vi "SutterController.vi"() -> ()   [LabVIEW 2012]
uses:
  <vilib>/Math Plots/3D Math Plots/3D Scatter/3D Scatter XCtrl/3D Scatter.xctl
  SerialController/Serial Controller.lvclass
  SerialController/Joystick.lvclass
  <vilib>/Utility/file.llb/Read From Spreadsheet File (DBL).vi
  <vilib>/Utility/file.llb/Write To Spreadsheet File (DBL).vi
panel:
  out "error out":errorcluster
  in  "Z limit":bool
  in  "TopLens":bool
  in  "overide":bool
  out "OutOfRange":bool
  in  "Set Maximum":bool
  in  "Set Minimum":bool
  out "positionLimits":dbl[][](array[numeric])
  out "Coarse":bool
  out "Locked":bool
  out "AxisStep":dbl[](array[numeric])
  out "ExternalInput":bool
  out "3D Scatter":refnum<class "3D Plot Datatype.lvclass">[](xcontrol)
  out "Moving":bool
  in  "stop":bool
  in  "Current Position":dbl[](array[numeric])
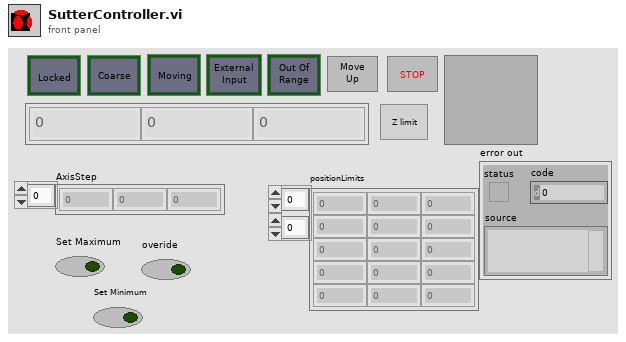
[diagram p1: front panel]
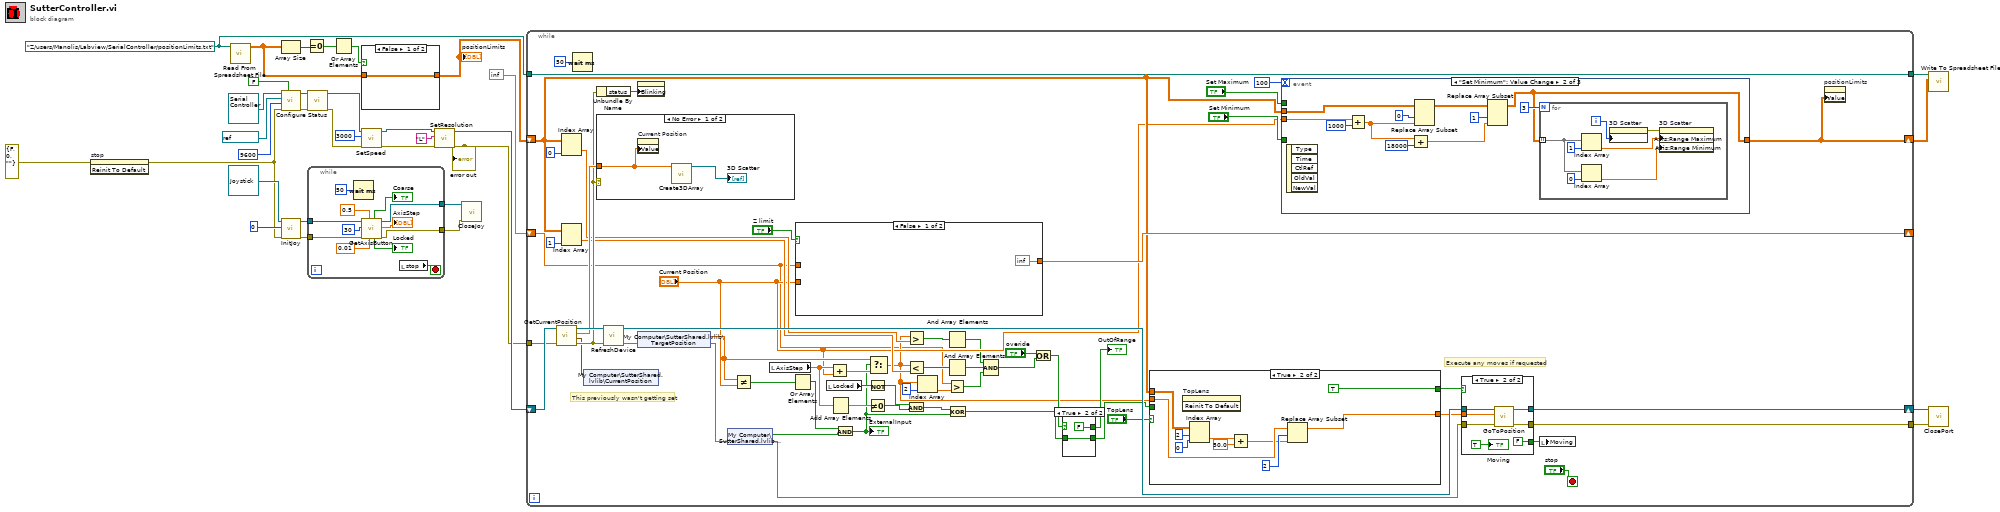
[diagram p0: block diagram]
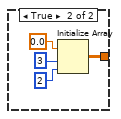
[diagram p2: hidden frame]
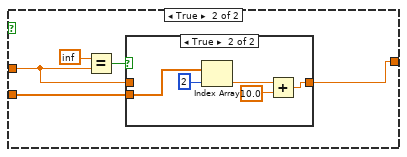
[diagram p3: hidden frame]
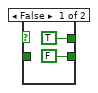
[diagram p6: hidden frame]
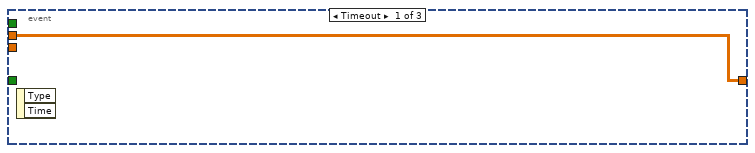
[diagram p7: hidden frame]
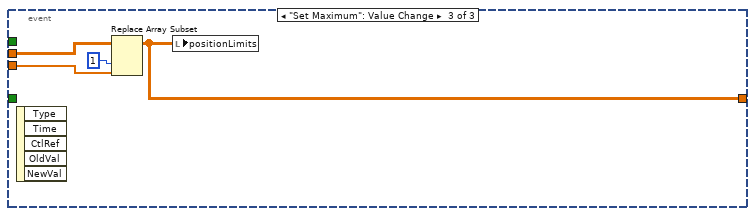
[diagram p8: hidden frame]
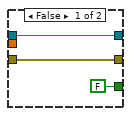
[diagram p9: hidden frame]
diagram:
  w10 = path "Z:/users/Manolis/Labview/SerialController/positionLimits.txt" ("Path")
  n1 = invoke on="stop" class="Bool (strict)" method="Reinit To Default"(error in=errorcluster {"status"=FALSE, "code"=0, "source"=""} ("error in (no error)")) -> (error out=w11:errorcluster)  [unwired: 2 in, 2 out]
  n2 = call-poly <vilib>:"Read From Spreadsheet File.vi"("file path (dialog if empty)"=w10) -> ("all rows"=w5:dbl[][])  [unwired: 6 in, 4 out]
  n3 = Array Size(array=w5) -> (size(s)=w7:i32[])
  n4 = call-dynamic "Configure.vi"("Reset"=FALSE, "error in (no error)"=w11, "baud rate (9600)"=u32 9600, "VISA resource name"=refnum<visa-resource-name> "COM6", "Serial Controller in"=refnum<class "Serial Controller.lvclass"> refnum) -> ("error out"=w32:errorcluster, "Serial Controller out"=w33:refnum<class "Serial Controller.lvclass">)  [unwired: 5 in]
  n5 = call-dynamic "InitJoy.vi"("error in (no error)"=w11, "device index"=0, "Joystick in"=refnum<class "Joystick.lvclass"> refnum) -> ("error out"=w15:errorcluster, "Joystick out"=w16:refnum<class "Joystick.lvclass">)  [unwired: 7 in]
  n6 = Equal To 0?(x=w7) -> (x = 0?=w6:bool[])
  n7 = call-dynamic "Status.vi"("error in (no error)"=w32, "Serial Controller in"=w33) -> ("error out"=w19:errorcluster, "Serial Controller out"=w21:refnum<class "Serial Controller.lvclass">)  [unwired: 7 in, 1 out]
  n8 = while {
    tunnel: w16 -> [w43]
    tunnel: w15 -> [w42]
    tunnel: [w40] -> w14
    tunnel: [w39] -> w13
    stop <- w45 stop-if-true
    n9 = Wait (ms)(milliseconds to wait=u32 50) -> ()  [unwired: 1 out]
    n10 = call-dynamic "GetAxisButton"("coarseFactor"=0.01, "fastFactor"=0.5, "error in (no error)"=w42, "timeout(s)"=u32 30, "Joystick in"=w43) -> ("error out"=w39:errorcluster, "AxisStep"=→"AxisStep":dbl[], "Joystick out"=w40:refnum<class "Joystick.lvclass">, "lock"=→"Locked":bool, "Coarse"=→"Coarse":bool)  [unwired: 2 in]
    n11 = local read "stop"() -> (w45:bool)
  }
  n12 = Or Array Elements(Boolean array=w6) -> (logical OR=w3:bool)
  n13 = case shown="False" w3 {
    tunnel: w5 -> [w46 _]
    tunnel: [w46 w47] -> w4
    frame False {
    }
    frame True {
      n14 = Initialize Array(0.0 ("element"), 3 ("dimension size"), 2 ("dimension size")) -> (w47:dbl[][])
    }
  }
  "positionLimits" <- w4
  n15 = call-dynamic "SetSpeed.vi"("error in (no error)"=w19, "Input: Speed in microns/sec"=3000, "Serial Controller in"=w21) -> ("error out"=w24:errorcluster, "Serial Controller out"=w23:refnum<class "Serial Controller.lvclass">)  [unwired: 5 in, 2 out]
  n16 = call-dynamic "SetResolution.vi"("error in (no error)"=w24, "Input: Resolution - H/L"="L", "Serial Controller in"=w23) -> ("error out"=w1:errorcluster, "Serial Controller out"=w20:refnum<class "Serial Controller.lvclass">)  [unwired: 7 in]
  "error out" <- w1
  n17 = call-dynamic "CloseJoy.vi"("error in (no error)"=w13, "Joystick in"=w14) -> ()  [unwired: 9 in, 1 out]
  n18 = while {
    shift-right: [w100] -> w27
    shift-left: w20 -> [w109]
    tunnel: [w89] -> w26
    tunnel: w1 -> [w95]
    tunnel: w10 -> [w80]
    tunnel: [w80] -> w9
    shift-right: [w65] -> w8
    shift-left: w4 -> [w62]
    shift-right: [w63] -> _
    shift-left: inf -> [w58]
    stop <- "stop" stop-if-true
    # "Execute any moves if requested"
    # "This previously wasn't getting set"
    n19 = call-dynamic "GetCurrentPosition.vi"("error in (no error)"=w95, "Serial Controller in"=w109) -> ("error out"=w105:errorcluster, "PositionBundle"=w52:cluster{"X":dbl, "Y":dbl, "Z":dbl, "Depth":dbl}, "Position"=w106:dbl[], "Serial Controller out"=w107:refnum<class "Serial Controller.lvclass">)  [unwired: 6 in]
    n20 = Index Array(array=w62, index (col)=0 ("disabled index (col)")) -> (element=w79:dbl[])  [unwired: 1 in]
    n21 = Index Array(array=w62, index (col)=1 ("disabled index (col)")) -> (element=w78:dbl[])  [unwired: 1 in]
    n22 = Wait (ms)(milliseconds to wait=u32 50) -> ()  [unwired: 1 out]
    n23 = shared-variable "My Computer\\SutterShared.lvlib\\CurrentPosition"(w52) -> ()  [unwired: 1 in, 1 out]
    n24 = Unbundle By Name(w105) -> ("status"=w103:bool)
    n25 = case shown="No Error" w105 {
      tunnel: w106 -> [w171 _]
      frame No Error {
        n26 = property on="Current Position" class="Arr (strict)"("Value"=w171) -> ()  [unwired: 2 in, 2 out]
        n27 = call "Create3DArray.vi"("Position"=w171) -> ("3D Plot lvclass Array out"=→"3D Scatter":refnum<class "3D Plot Datatype.lvclass">[])  [unwired: 10 in]
      }
      frame Error {
      }
    }
    n28 = call-dynamic "RefreshDevice.vi"("error in (no error)"=w105, "Serial Controller in"=w107) -> ("error out"=w94:errorcluster, "Serial Controller out"=w96:refnum<class "Serial Controller.lvclass">)  [unwired: 8 in]
    n29 = property on="Current Position" class="Arr (strict)"("Blinking"=w103) -> ()  [unwired: 2 in, 2 out]
    n30 = shared-variable "My Computer\\SutterShared.lvlib\\TargetPosition"(error in=w94) -> (w92:dbl[], error out=w88:errorcluster)
    n31 = shared-variable "My Computer\\SutterShared.lvlib\\Move"(error in=w88) -> (w85:bool, error out=w87:errorcluster)
    n32 = Not Equal?(x=w92, y="Current Position") -> (x != y?=w93:bool[])
    n33 = local read "AxisStep"() -> (w102:dbl[])
    n34 = Or Array Elements(Boolean array=w93) -> (logical OR=w86:bool)
    n35 = case shown="False" "Z limit" {
      tunnel: w58 -> [_ w111]
      tunnel: [inf w114] -> w63
      tunnel: "Current Position" -> [_ w115]
      frame False {
      }
      frame True {
        n36 = Equal?(x=inf, y=w111) -> (x = y?=w112:bool)
        n37 = case shown="True" w112 {
          tunnel: w115 -> [_ w121]
          tunnel: [w116 w118] -> w114
          tunnel: w111 -> [w116 _]
          frame False {
          }
          frame True {
            n38 = Index Array(array=w121, index=2) -> (element=w119:dbl)
            n39 = Add(x=w119, y=10.0) -> (x+y=w118:dbl)
          }
        }
      }
    }
    n40 = local read "Locked"() -> (w98:bool)
    n41 = Add(x=w102, y="Current Position") -> (x+y=w91:dbl[])
    n42 = Add Array Elements(numeric array=w102) -> (sum=w101:dbl)
    n43 = And(x=w86, y=w85) -> (x .and. y?=w84:bool)
    "ExternalInput" <- w84
    n44 = Not(x=w98) -> (.not. x?=w97:bool)
    n45 = Not Equal To 0?(x=w101) -> (x != 0?=w99:bool)
    n46 = Select(t=w92, s=w84, f=w91) -> (s? t:f=w60:dbl[])
    n47 = Greater?(x=w60, y=w79) -> (0:w75:bool[])
    n48 = Less?(x=w60, y=w78) -> (x < y?=w74:bool[])
    n49 = And(x=w97, y=w99) -> (x .and. y?=w90:bool)
    n50 = Index Array(array=w60, index=2) -> (element=w57:dbl)
    n51 = And Array Elements(Boolean array=w75) -> (logical AND=w56:bool)
    n52 = And Array Elements(Boolean array=w74) -> (logical AND=w55:bool)
    n53 = Greater?(x=w58, y=w57) -> (0:w53:bool)
    n54 = Exclusive Or(1:w84, 2:w90) -> (0:w72:bool)
    n55 = Compound Arithmetic op=AND(w56, w55, w53) -> (w54:bool)
    n56 = Or(x="overide", y=w54) -> (x .or. y?=w71:bool)
    n57 = case shown="True" w71 {
      tunnel: w72 -> [_ w137]
      tunnel: [FALSE w137] -> w68
      tunnel: [TRUE FALSE] -> w73
      frame False {
      }
      frame True {
      }
    }
    "OutOfRange" <- w73
    n58 = case shown="True" "TopLens" {
      tunnel: w68 -> [w123 _]
      tunnel: [w123 TRUE] -> w67
      tunnel: w60 -> [w122 w132]
      tunnel: [w122 w130] -> w66
      tunnel: w62 -> [_ w129]
      frame False {
      }
      frame True {
        n59 = invoke on="TopLens" class="Bool (strict)" method="Reinit To Default"() -> ()  [unwired: 3 in, 3 out]
        n60 = Index Array(array=w129, index (row)=2 ("disabled index (row)"), index (col)=0 ("disabled index (col)")) -> (element=w126:dbl)
        n61 = Add(x=w126, y=50.0) -> (x+y=w125:dbl)
        n62 = Replace Array Subset(array=w132, new element=w125, index=2) -> (w130:dbl[])
      }
    }
    n63 = event shown="[1] \"Set Minimum\": Value Change" {
      selector: _ -> [_ _ _]
      dyn-events: _ -> [_ _ _]
      timeout: 100 -> [_ _ _]
      tunnel: "Set Minimum" -> [_ _ _]
      tunnel: "Current Position" -> [_ w147 w160]
      tunnel: w62 -> [w138 w149 w159]
      tunnel: "Set Maximum" -> [_ _ _]
      tunnel: [w138 w139 w157] -> w65
      event Timeout {
        n64 = event-data() -> ()  [unwired: 1 in, 2 out]
      }
      event "Set Minimum": Value Change {
        n65 = event-data() -> ()  [unwired: 1 in, 5 out]
        n66 = Add(x=w147, y=1000) -> (x+y=w143:dbl[])
        n67 = Add(x=w143, y=18000) -> (x+y=w142:dbl[])
        n68 = Replace Array Subset(array=w149, new element=w143, index (col)=0 ("disabled index (col)")) -> (w144:dbl[][])  [unwired: 1 in]
        n69 = Replace Array Subset(array=w144, new element=w142, index (col)=1 ("disabled index (col)")) -> (w139:dbl[][])  [unwired: 1 in]
        n70 = for {
          N: 3 -> [_]
          tunnel: w139 -> [w155] mode=indexing
          i -> [w156]
          n71 = Index Array(array=w155, index=1) -> (element=w153:dbl)
          n72 = Index Array(array=w155, index=0) -> (element=w154:dbl)
          n73 = property on="3D Scatter" class="3D Scatter (strict)"("Axis:Active Axis"=w156) -> (error out=w150:errorcluster)  [unwired: 2 in, 1 out]
          n74 = property on="3D Scatter" class="3D Scatter (strict)"(error in=w150, "Axis:Range Maximum"=w153, "Axis:Range Minimum"=w154) -> ()  [unwired: 1 in, 2 out]
        }
      }
      event "Set Maximum": Value Change {
        n75 = event-data() -> ()  [unwired: 1 in, 5 out]
        n76 = Replace Array Subset(array=w159, new element=w160, index (col)=1 ("disabled index (col)")) -> (w157:dbl[][])  [unwired: 1 in]
        n77 = local write "positionLimits"(w157) -> ()
      }
    }
    n78 = case shown="True" w67 {
      tunnel: w96 -> [w163 w170]
      tunnel: [w163 w166] -> w100
      tunnel: w87 -> [w162 w169]
      tunnel: [w162 w165] -> w89
      tunnel: w66 -> [_ w168]
      tunnel: [FALSE FALSE] -> w51
      frame False {
      }
      frame True {
        n79 = call-dynamic "GoToPosition.vi"("error in (no error)"=w169, "Position"=w168, "Serial Controller in"=w170) -> ("error out"=w165:errorcluster, "Serial Controller out"=w166:refnum<class "Serial Controller.lvclass">)  [unwired: 6 in, 1 out]
        "Moving" <- TRUE ("Boolean")
      }
    }
    n80 = local write "Moving"(w51) -> ()
    n81 = property on="positionLimits" class="Arr (strict)"("Value"=w65) -> ()  [unwired: 2 in, 2 out]
  }
  n82 = call-poly <vilib>:"Write To Spreadsheet File.vi"("2D data"=w8, "file path (dialog if empty)"=w9) -> ()  [unwired: 6 in, 1 out]
  n83 = call-dynamic "ClosePort.vi"("error in (no error)"=w26, "Serial Controller in"=w27) -> ()  [unwired: 9 in, 1 out]
